vi "Read Incoming Bytes.vi"(8 "error in (no error)":errorcluster, 9 "timeout (1000 ms)":i32=1000, 10 "bytes to read (100)":i32=100, 11 "Connection.TCP-TLS in":refnum<class "Connection.TCP-TLS.lvclass">) -> (0 "error out":errorcluster, 1 "timed out":bool, 2 "Bytes":u8[](array[numeric]) format="%08b", 3 "Connection.TCP-TLS out":refnum<class "Connection.TCP-TLS.lvclass">, 4 "connected":bool)   [LabVIEW 2020]
uses:
  Connection.TCP-TLS.lvclass
  Connection.TCP-TLS.lvclass/Connection.TCP-TLS.ctl
  C:/Program Files (x86)/National Instruments/LabVIEW 2020/vi.lib/LabVIEW Open Source Project/MQTT TCP Connection/MQTT_TCP/Connection/TCPConnection.lvclass
  C:/Program Files (x86)/National Instruments/LabVIEW 2020/vi.lib/LabVIEW Open Source Project/MQTT Connection/MQTT_Connection/Connection/Connection.lvclass
  C:/Projects/LVOS/MQTT-Connection-TCP.TLS/source/Connection.SecuredTCP/Connection.TCP-TLS.lvclass
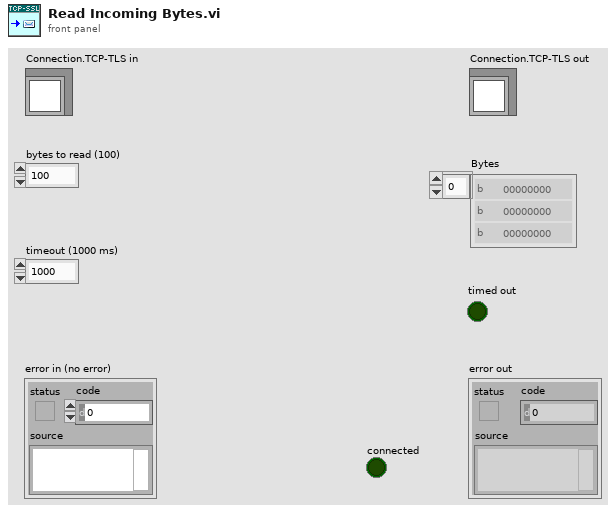
[diagram p1: front panel]
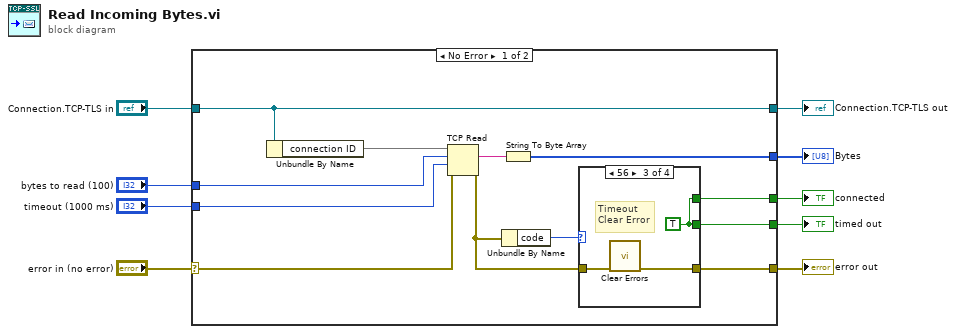
[diagram p0: block diagram]
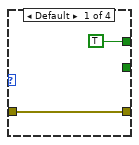
[diagram p2: hidden frame]
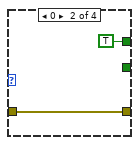
[diagram p3: hidden frame]
diagram:
  n1 = case shown="No Error" "error in (no error)" {
    selector: "error in (no error)" -> [w20 w31]
    tunnel: [w11 w31] -> w3
    tunnel: [w12 w30] -> w5
    tunnel: "Connection.TCP-TLS in" -> [w12 w30]
    tunnel: [w18 _] -> w4
    tunnel: "bytes to read (100)" -> [w15 _]
    tunnel: "timeout (1000 ms)" -> [w14 _]
    tunnel: [w13 _] -> w1
    tunnel: [w10 _] -> w2
    frame No Error {
      n2 = Unbundle By Name(w12) -> ("connection ID"=w21)
      n3 = TCP Read(connection ID=w21, bytes to read=w15, error in (no error)=w20, 9:w14) -> (data out=w19:string, error out=w16:errorcluster)  [unwired: 1 in, 1 out]
      n4 = Unbundle By Name(w16) -> ("code"=w17:i32)
      n5 = String To Byte Array(string=w19) -> (unsigned byte array=w18:u8[])
      n6 = case shown="56" w17 {
        tunnel: [w23 w25 w28 w29] -> w11
        tunnel: w16 -> [w23 w25 w27 w29]
        tunnel: [_ _ w26 _] -> w13
        tunnel: [TRUE TRUE w26 _] -> w10
        frame Default {
        }
        frame 0 {
        }
        frame 56 {
          w26 = TRUE
          # "Timeout\nClear Error"
          n7 = call <vilib>:"Clear Errors.vi"("error in (no error)"=w27) -> ("error out"=w28:errorcluster)  [unwired: 5 in, 1 out]
        }
        frame 66 {
          # "Disconnection\nby peer"
        }
      }
    }
    frame Error {
    }
  }
  "error out" <- w3
  "Connection.TCP-TLS out" <- w5
  "Bytes" <- w4
  "timed out" <- w1
  "connected" <- w2
